vi "Socket_Get EOLData.vi"(11 "station name":string) -> (3 "data out":string[](array[string]))   [LabVIEW 2015]
uses:
  Ctldef/Socket_EOLData.ctl
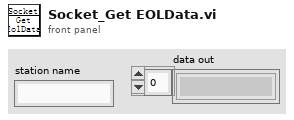
[diagram p1: front panel]
types:
  T1 = enum16{"Read", "Write", "ReadWrite", "BufferedRead", "BufferedReadWrite"}
  T2 = typedef "Socket_EOLData.ctl" = cluster{"ST55":string[][], "ST80":string[][], "ST90":string[][], "ST100":string[][], "ST110":string[][]}
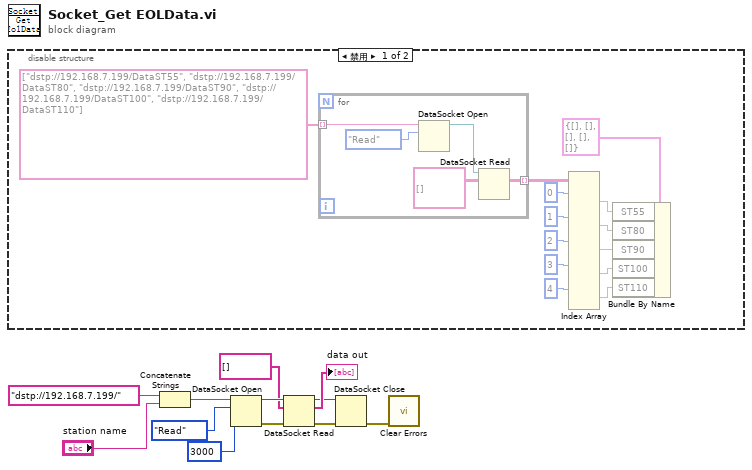
[diagram p0: block diagram]
diagram:
  n1 = disable-structure shown="禁用" {
    frame Disabled {
      n2 = for {
        tunnel: string[] ["dstp://192.168.7.199/DataST55", "dstp://192.168.7.199/DataST80", "dstp://192.168.7.199/DataST90", "dstp://192.168.7.199/DataST100", "dstp://192.168.7.199/DataST110"] -> [w27] mode=indexing
        tunnel: [w26] -> w24 mode=indexing
        n3 = DataSocket Open(10:T1."Read" ("模式"), 11:w27) -> (3:w29:refnum<k13>)  [unwired: 2 in, 1 out]
        n4 = DataSocket Read(10:string[][] [], 11:w29) -> (2:w26:string[][])  [unwired: 3 in, 6 out]
      }
      n5 = Index Array(array=w24, index (dim 0) #1=0 ("索引 (页)"), index (dim 0) #2=1 ("索引 (页)"), index (dim 0) #3=2 ("索引 (页)"), index (dim 0) #4=3 ("索引 (页)"), index (dim 0) #5=4 ("索引 (页)")) -> (element #1=w17:string[][], element #2=w13:string[][], element #3=w14:string[][], element #4=w15:string[][], element #5=w16:string[][])  [unwired: 10 in]
      n6 = Bundle By Name(cluster=T2 {"ST55"=[], "ST80"=[], "ST90"=[], "ST100"=[], "ST110"=[]} ("Socket_EOLData"), "ST55"=w17, "ST80"=w13, "ST90"=w14, "ST100"=w15, "ST110"=w16) -> ()  [unwired: 1 out]
    }
    frame Enabled {
    }
  }
  n7 = Concatenate Strings("dstp://192.168.7.199/" ("URL"), "station name") -> (w9:string)
  n8 = DataSocket Open(9:3000 ("毫秒超时(10000)"), 10:T1."Read" ("模式"), 11:w9) -> (0:w3:errorcluster, 3:w8:refnum<k13>)  [unwired: 1 in]
  n9 = DataSocket Read(8:w3, 10:string[] [], 11:w8) -> (0:w4:errorcluster, 2:→"data out":string[], 3:w5:refnum<k13>)  [unwired: 2 in, 4 out]
  n10 = DataSocket Close(8:w4, 11:w5) -> (0:w2:errorcluster)  [unwired: 1 in, 1 out]
  n11 = call <vilib>:"Clear Errors.vi"("error in (no error)"=w2) -> ()  [unwired: 5 in, 2 out]
